vi "Theory.vi"(10 "Input":string) -> (0 "error out":errorcluster)   [LabVIEW 2017, in "LVUnitTestBuilder.Tests.lvlib" / "LibraryWithTheory.lvlib"]
uses:
  LibraryWithTheory.lvlib
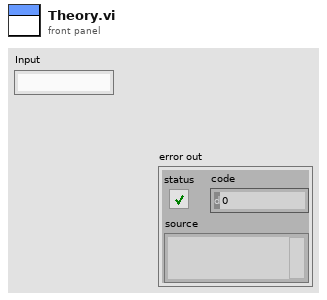
[diagram p1: front panel]
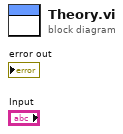
[diagram p0: block diagram]
diagram:
